vi "produceTimingTicks.vi"(8 "error in (no error)":errorcluster, 10 "Channel":refnum<class "Channel.lvclass">, 11 "ScriptEvent in":refnum<class "ScriptEvent.lvclass">) -> (0 "error out":errorcluster, 2 "timingTick":refnum<class "ScriptEventList.lvclass">, 3 "ScriptEvent out":refnum<class "ScriptEvent.lvclass">)   [LabVIEW 2011, in "Tools.lvlib" / "Scripting.lvlib" / "ScriptEvent.lvclass"]
uses:
  ScriptEvent.lvclass
  DatabaseHelpers/Database Objects/Channel/Channel.lvclass
  ScriptEventList/ScriptEventList.lvclass
  ScriptEvent.lvclass/ScriptEvent.ctl
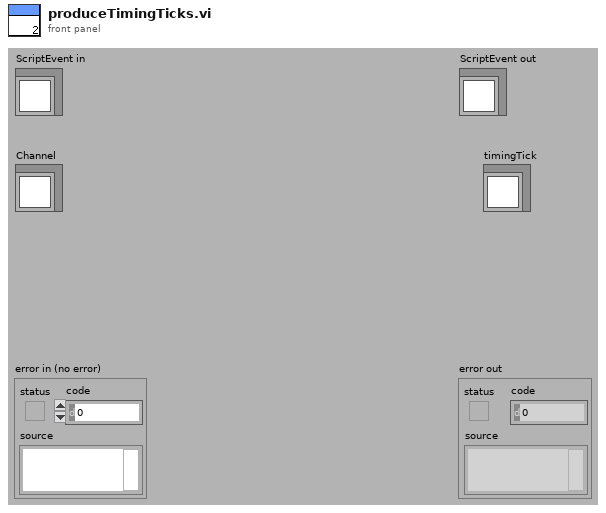
[diagram p1: front panel]
types:
  T1 = enum16{"changeValue", "pulse", "clock", "rampUp", "rampDown", "singleTone", "singleToneRamp", "playFile"}
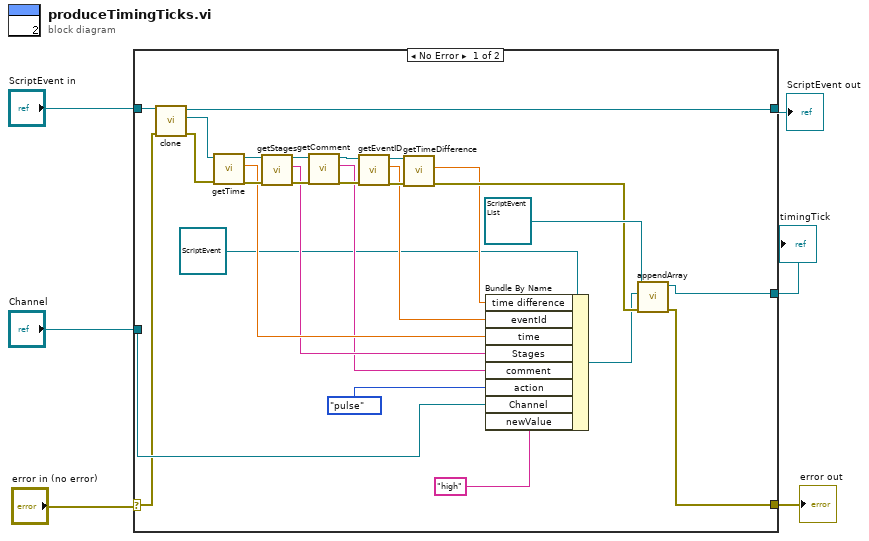
[diagram p0: block diagram]
diagram:
  n1 = case shown="No Error" "error in (no error)" {
    selector: "error in (no error)" -> [w26 w35]
    tunnel: [w29 w35] -> w6
    tunnel: [w27 w34] -> w4
    tunnel: "ScriptEvent in" -> [w28 w34]
    tunnel: "Channel" -> [w33 _]
    tunnel: [w31 _] -> w1
    frame No Error {
      n2 = call-dynamic "clone.vi"("error in (no error)"=w26, "ScriptEvent in"=w28) -> ("error out"=w15:errorcluster, "clone"=w16:refnum<class "ScriptEvent.lvclass">, "ScriptEvent out"=w27:refnum<class "ScriptEvent.lvclass">)  [unwired: 7 in]
      n3 = call "getTime.vi"("error in (no error)"=w15, "ScriptEvent.lvclass in"=w16) -> ("error out"=w24:errorcluster, "time"=w11:dbl, "ScriptEvent.lvclass out"=w23:refnum<class "ScriptEvent.lvclass">)  [unwired: 7 in]
      n4 = call "getStages.vi"("error in (no error)"=w24, "ScriptEvent.lvclass in"=w23) -> ("error out"=w22:errorcluster, "Stage"=w10:string, "ScriptEvent.lvclass out"=w21:refnum<class "ScriptEvent.lvclass">)  [unwired: 7 in]
      n5 = call "getComment.vi"("error in (no error)"=w22, "ScriptEvent.lvclass in"=w21) -> ("error out"=w19:errorcluster, "comment"=w9:string, "ScriptEvent.lvclass out"=w20:refnum<class "ScriptEvent.lvclass">)  [unwired: 7 in]
      n6 = call "getEventID.vi"("error in (no error)"=w19, "ScriptEvent in"=w20) -> ("error out"=w18:errorcluster, "eventId"=w12:dbl, "ScriptEvent out"=w17:refnum<class "ScriptEvent.lvclass">)  [unwired: 7 in]
      n7 = call "getTimeDifference.vi"("error in (no error)"=w18, "ScriptEvent.lvclass in"=w17) -> ("error out"=w14:errorcluster, "time difference"=w13:dbl)  [unwired: 7 in, 1 out]
      n8 = Bundle By Name(cluster=refnum<class "ScriptEvent.lvclass"> refnum ("Tools.lvlib:Scripting.lvlib:ScriptEvent.lvclass"), "time difference"=w13, "eventId"=w12, "time"=w11, "Stages"=w10, "comment"=w9, "action"=T1."pulse", "Channel"=w33, "newValue"="high") -> (w7:refnum<class "ScriptEvent.lvclass">)
      n9 = call "appendArray.vi"("error in (no error)"=w14, "ScriptEvent"=w7, "ScriptEventList in"=refnum<class "ScriptEventList.lvclass"> refnum) -> ("error out"=w29:errorcluster, "ScriptEventList out"=w31:refnum<class "ScriptEventList.lvclass">)  [unwired: 6 in, 1 out]
    }
    frame Error {
    }
  }
  "error out" <- w6
  "ScriptEvent out" <- w4
  "timingTick" <- w1
